vi "Adjust Limbus.vi"(8 "error in (no error)":errorcluster, 9 "Results":T4, 10 "Treatment":T2, 11 "Images":T3) -> (0 "error out":errorcluster, 1 "Results":T4, 2 "Treatment":T2, 3 "Images":T3)   [LabVIEW 2015]
uses:
  controls/Results.ctl
  controls/Treatment Parameters.ctl
  controls/Images.ctl
  <vilib>/vision/Image Controls.llb/IMAQ Image.ctl
panel:
  out "Image 2":T1(plugin-control)
  out "Image":T1(plugin-control)
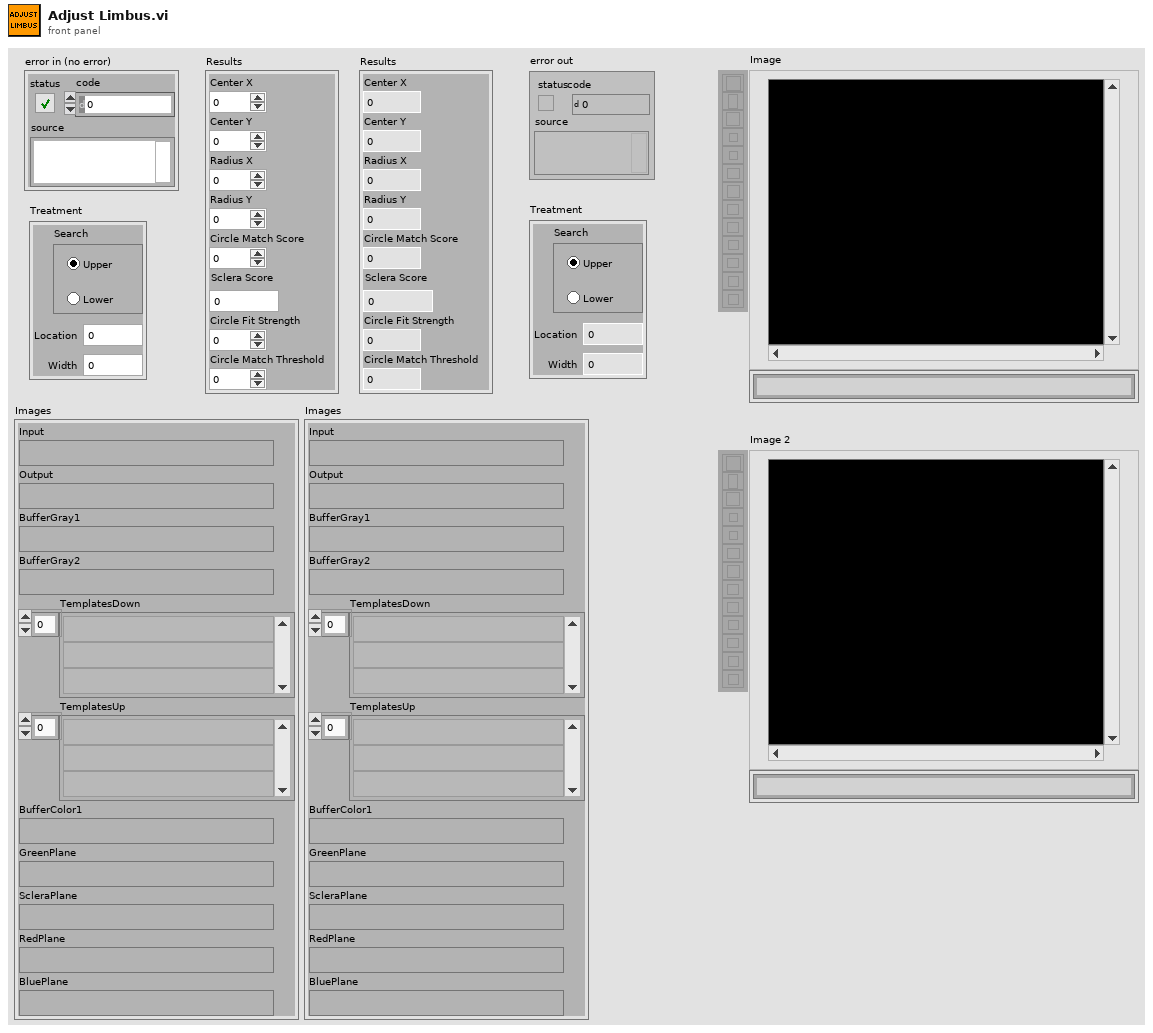
[diagram p1: front panel]
types:
  T1 = typedef "IMAQ Image.ctl" = refnum<image>
  T2 = typedef "Treatment Parameters.ctl" = cluster{"Location":dbl, "Width":dbl, "Search":enum32{"Upper", "Lower"}}
  T3 = typedef "Images.ctl" = cluster{"Input":T1, "Output":T1, "BufferGray1":T1, "BufferGray2":T1, "TemplatesDown":T1[], "TemplatesUp":T1[], "BufferColor1":T1, "GreenPlane":T1, "ScleraPlane":T1, "RedPlane":T1, "BluePlane":T1}
  T4 = typedef "Results.ctl" = cluster{"Center X":i32, "Center Y":i32, "Radius X":i32, "Radius Y":i32, "Circle Match Score":i32, "Sclera Score":dbl, "Circle Fit Strength":i32, "Circle Match Threshold":i32}
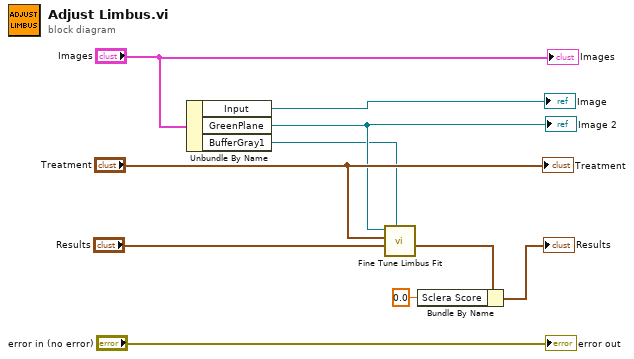
[diagram p0: block diagram]
diagram:
  n1 = Unbundle By Name("Images") -> ("Input"=→"Image":T1, "GreenPlane"=w2:T1, "BufferGray1"=w1:T1)
  "Image 2" <- w2
  n2 = call "Fine Tune Limbus Fit.vi"("Grayscale Buffer 1"=w1, "Results"="Results", "Treatment"="Treatment", "Green Plane"=w2) -> ("Results out"=w4:T4)  [unwired: 6 in, 1 out]
  n3 = Bundle By Name(cluster=w4, "Sclera Score"=0.0 ("Sclera Ratio")) -> (→"Results":T4)
  "Images" <- "Images"
  "Treatment" <- "Treatment"
  "error out" <- "error in (no error)"
